vi "Spam - Generate Errors.vi"(8 "Error In":errorcluster, 11 "Variant":variant) -> (0 "Error Out":errorcluster)   [LabVIEW 2023, in "Anti-Spam Tester (AST).lvlib"]
doc: "Blank VI with error handling."
uses:
  Anti-Spam Tester (AST).lvlib
  Error Manager/Error Manager.lvlib
panel:
  out "Number of errors":i32
  out "Errors":errorcluster[](array[cluster])
  # "Input\nInputs to the VI"
  # "Development\nControls or indicators that are useful for development or testing, but which are not outputs of the VI."
  # "Output\nOutputs of the VI"
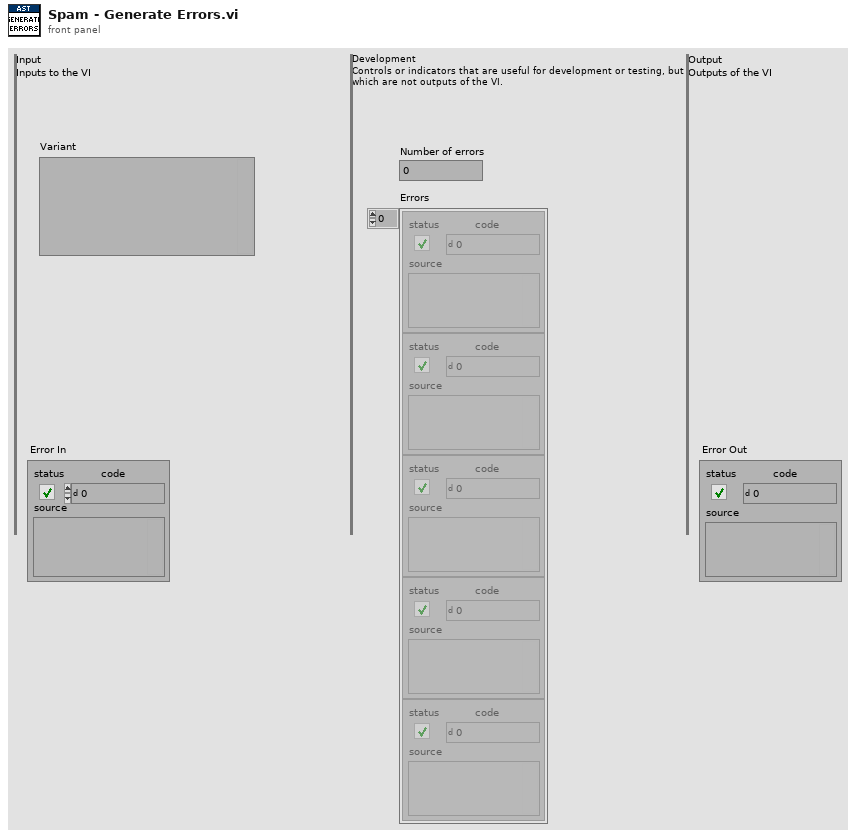
[diagram p1: front panel]
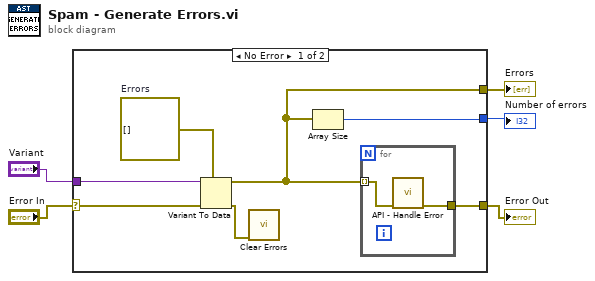
[diagram p0: block diagram]
diagram:
  n1 = case shown="No Error" "Error In" {
    selector: "Error In" -> [w12 w15]
    tunnel: "Variant" -> [w9 _]
    tunnel: [w8 w15] -> w3
    tunnel: [w7 _] -> w2
    tunnel: [w6 _] -> w1
    frame No Error {
      w10 = errorcluster[] []  # Errors
      n2 = Variant To Data(error in=w12, type=w10, Variant=w9) -> (data=w7:errorcluster[], error out=w11:errorcluster)
      n3 = call <vilib>:"Clear Errors.vi"("error in (no error)"=w11) -> ()  [unwired: 5 in, 2 out]
      n4 = Array Size(array=w7) -> (size(s)=w6:i32)
      n5 = for {
        tunnel: w7 -> [w13] mode=indexing
        tunnel: [w14] -> w8
        n6 = call "API - Handle Error.vi"("error in"=w13) -> ("error out"=w14:errorcluster)  [unwired: 10 in]
      }
    }
    frame Error {
    }
  }
  "Error Out" <- w3
  "Errors" <- w2
  "Number of errors" <- w1
